vi "Create StringMap.vi"(5 "StringMap in":refnum<class "StringMap.lvclass">, 7 "Map Implementation (Variant Attributes)":refnum<class "MapImp.lvclass">, 8 "error in (no error)":errorcluster) -> (0 "error out":errorcluster, 3 "StringMap out":refnum<class "StringMap.lvclass">)   [LabVIEW 2013, in "LapDog.Collections.v_.Maps.lvlib" / "StringMap.lvclass"]
uses:
  StringMap.lvclass
  ObjectMap/ObjectMap.lvclass
  MapImp/MapImp.lvclass
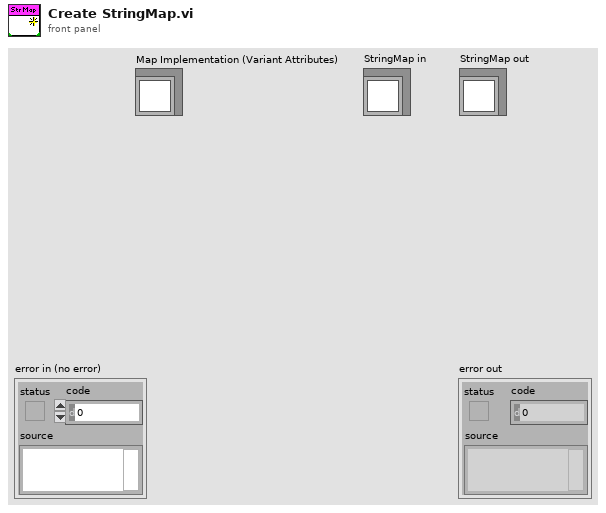
[diagram p1: front panel]
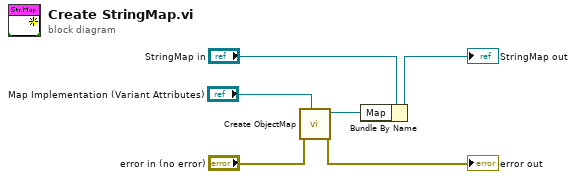
[diagram p0: block diagram]
diagram:
  n1 = call "Create ObjectMap.vi"("Map Implementation (Variant Attributes)"="Map Implementation (Variant Attributes)", "error in (no error)"="error in (no error)") -> ("error out"=→"error out":errorcluster, "ObjectMap"=w1:refnum<class "ObjectMap.lvclass">)  [unwired: 8 in]
  n2 = Bundle By Name(cluster="StringMap in", "Map"=w1) -> (→"StringMap out":refnum<class "StringMap.lvclass">)
